vi "Agilent VNA Wait for Operation Complete (OPC).vi"(7 "Agilent VNA":T1, 8 "error in (no error)":errorcluster, 9 "Timeout, ms (10000)":u32=10000, 11 "VISA Resource Name":refnum<visa-resource-name>) -> (0 "error out":errorcluster, 3 "dup VISA Resource Name":refnum<visa-resource-name>)   [LabVIEW 2011]
uses:
  TypeDefs/Agilent VNA Instrument Info.ctl
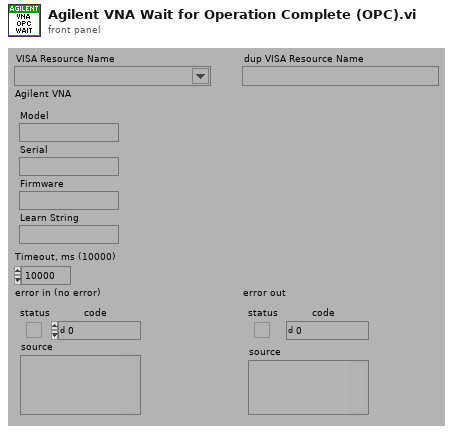
[diagram p1: front panel]
types:
  T1 = typedef "Agilent VNA Instrument Info.ctl" = cluster{"Model":string, "Serial":string, "Firmware":string, "Learn String":string}
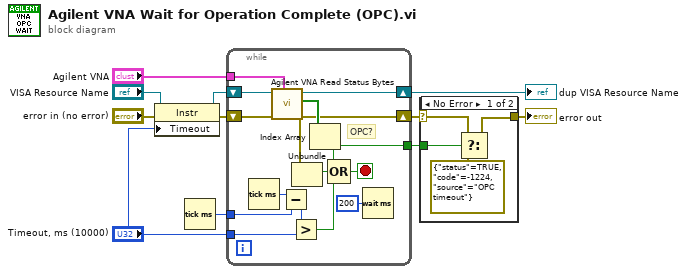
[diagram p0: block diagram]
diagram:
  n1 = property class="Instr"(reference="VISA Resource Name", error in="error in (no error)", "Timeout"="Timeout, ms (10000)") -> (reference out=w4:refnum<visa-resource-name>, error out=w2:errorcluster)
  n2 = Tick Count (ms)() -> (millisecond timer value=w11:u32)
  n3 = while {
    tunnel: [w14] -> w10
    tunnel: "Timeout, ms (10000)" -> [w23]
    tunnel: w11 -> [w26]
    shift-right: [w18] -> w9
    shift-left: w2 -> [w19]
    shift-right: [w13] -> w7
    shift-left: w4 -> [w21]
    tunnel: "Agilent VNA" -> [w12]
    stop <- w15 stop-if-true
    # "OPC?"
    n4 = Tick Count (ms)() -> (millisecond timer value=w25:u32)
    n5 = call "Agilent VNA Read Status Bytes.vi"("Agilent VNA"=w12, "error in (no error)"=w19, "VISA Resource Name"=w21) -> ("error out"=w18:errorcluster, "Event Status Register"=w20:bool[], "dup VISA Resource Name"=w13:refnum<visa-resource-name>)  [unwired: 1 in, 5 out]
    n6 = Subtract(x=w25, y=w26) -> (x-y=w24:u32)
    n7 = Greater?(x=w24, y=w23) -> (0:w16:bool)
    n8 = Unbundle(w18) -> ("status"=w17:bool)  [unwired: 2 out]
    n9 = Index Array(array=w20) -> (element=w14:bool)  [unwired: 1 in]
    n10 = Compound Arithmetic op=OR(w14, w17, w16) -> (w15:bool)
    n11 = Wait (ms)(milliseconds to wait=u32 200) -> ()  [unwired: 1 out]
  }
  "dup VISA Resource Name" <- w7
  n12 = case shown="No Error" w9 {
    selector: w9 -> [w29 w31]
    tunnel: w10 -> [w30 _]
    tunnel: [w28 w31] -> w8
    frame No Error {
      n13 = Select(t=w29, s=w30, f=errorcluster {"status"=TRUE, "code"=-1224, "source"="OPC timeout"}) -> (s? t:f=w28:errorcluster)
    }
    frame Error {
    }
  }
  "error out" <- w8
